vi "Is Channel Name Existing.vi"(8 "error in (no error)":errorcluster, 9 "Channel Name":string, 10 "Group Name":string, 11 "TDMS File Ref In":refnum<k34>) -> (0 "error out":errorcluster, 2 "Existed?":bool, 3 "TDMS File Ref Out":refnum<k34>)   [LabVIEW 2013, in "Agilent 90000 Series.lvlib"]
doc: "Checks whether the channel name is already existing in the TDMS file."
uses:
  Agilent 90000 Series.lvlib
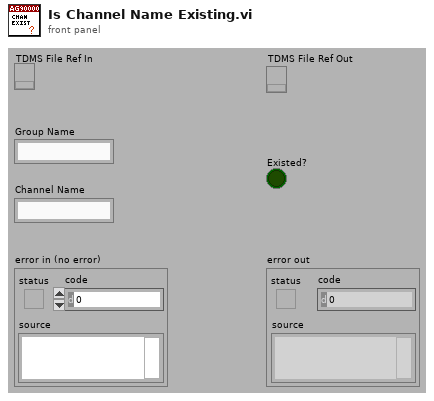
[diagram p1: front panel]
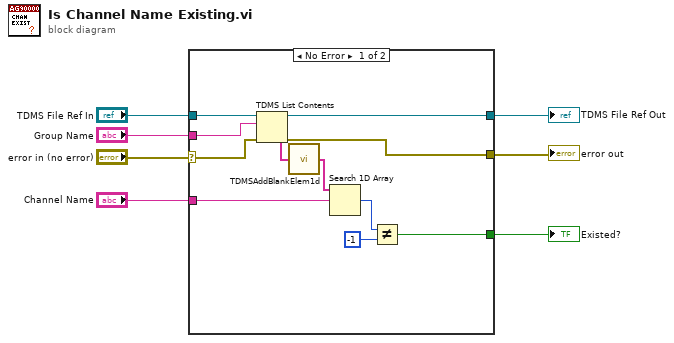
[diagram p0: block diagram]
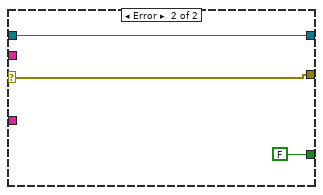
[diagram p2: hidden frame]
diagram:
  n1 = case shown="No Error" "error in (no error)" {
    selector: "error in (no error)" -> [w15 w20]
    tunnel: "Group Name" -> [w18 _]
    tunnel: "TDMS File Ref In" -> [w17 w21]
    tunnel: [w16 w21] -> w5
    tunnel: [w14 w20] -> w3
    tunnel: "Channel Name" -> [w12 _]
    tunnel: [w9 FALSE] -> w1
    frame No Error {
      n2 = TDMS List Contents(4:w15, 6:w18, 7:w17) -> (0:w14:errorcluster, 1:w8:string[], 3:w16:refnum<k34>)  [unwired: 1 out]
      n3 = call <vilib>:"TDMSAddBlankElem1d.vi"("input string array"=w8) -> ("output string array with blank element at the beginning"=w13:string[])
      n4 = Search 1D Array(1D array=w13, element=w12) -> (index of element=w11:i32)  [unwired: 1 in]
      n5 = Not Equal?(x=w11, y=-1) -> (x != y?=w9:bool)
    }
    frame Error {
    }
  }
  "TDMS File Ref Out" <- w5
  "error out" <- w3
  "Existed?" <- w1
